vi "Teleop.vi"(10 "Match Info":T2={"Autonomous Elapsed Seconds"=0.0, "TeleOp Elapsed Seconds"=0.0, "Disabled Elapsed Seconds"=0.0, "Visited Autonomous"=FALSE, "Visited TeleOp"=FALSE, "Visited Disabled"=FALSE, "Autonomous Settings"={"Autonomous Style"=enum."Independent", "VI Refnum"=refnum}}, 11 "Call Context":T3) -> ()   [LabVIEW 2017]
doc: "This VI is called for each enabled TeleOp packet received from the DS. It is typically used to read from joysticks and other inputs and update I/O or setpoints for timed control loops. It should complete and return within 20 milliseconds or risk missing DS packets."
uses:
  <vilib>/Rock Robotics/WPI/DriverStation/WPI_DriverStationDerivedRobotMode.ctl
  <vilib>/Rock Robotics/WPI/DriverStation/WPI_DriverStationMatch Info.ctl
  Framework/Robot Global Data.vi
panel:
  in  "Tab Control":T1(tab)
  out "X_AxisCmd":dbl(graph)
  out "Y_AxisCmd":dbl(graph)
  out "RotationCmd":dbl(graph)
  out "DriveMotors":dbl[](graph)
  out "LiftMotorCmd":dbl(graph)
  out "ArmLiftMotorCmd":dbl(graph)
  out "Lift Max Limit":bool
  out "Lift Min Limit":bool
  out "Arm Lift Max Limit":bool
  out "Arm Lift Min Limit":bool
  out "RightArmMotorCmd":dbl(graph)
  out "LeftArmMotorCmd":dbl(graph)
  out "Right Arm Max Limit":bool
  out "Right Arm Min Limit":bool
  out "Left Arm Max Limit":bool
  out "Left Arm Min Limit":bool
  out "SqueezeMotorCmd":dbl(graph)
  out "HandMotorsCmd":dbl(graph)
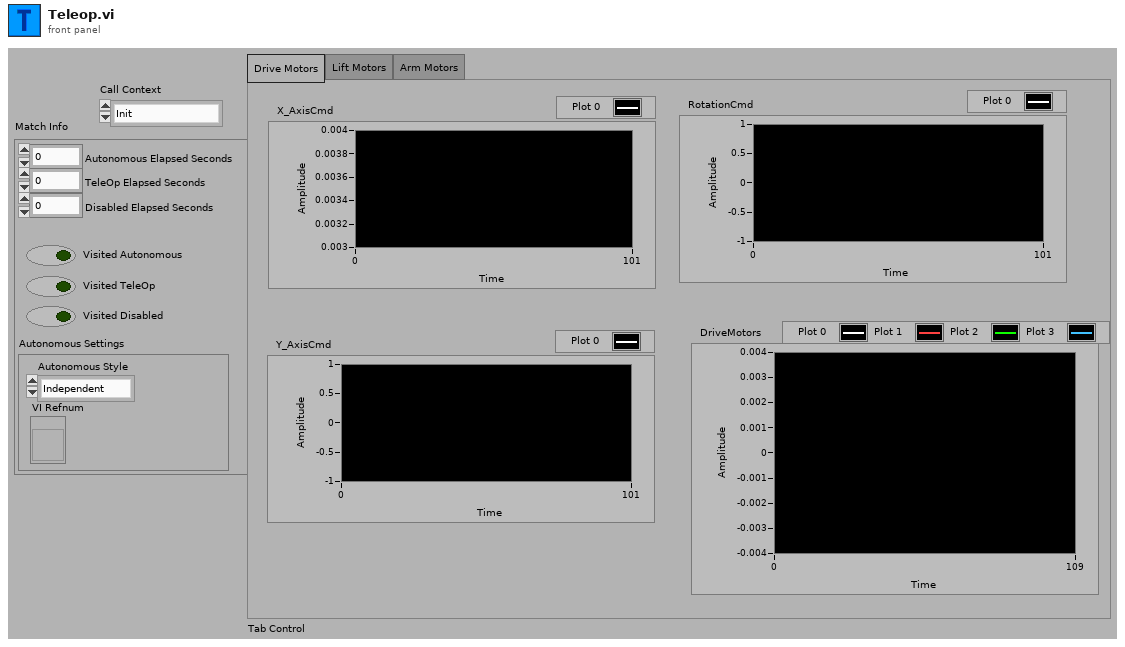
[diagram p1: front panel]
types:
  T1 = enum32{"Drive Motors", "Lift Motors", "Arm Motors"}
  T2 = typedef "WPI_DriverStationMatch Info.ctl" = cluster{"Autonomous Elapsed Seconds":dbl, "TeleOp Elapsed Seconds":dbl, "Disabled Elapsed Seconds":dbl, "Visited Autonomous":bool, "Visited TeleOp":bool, "Visited Disabled":bool, "Autonomous Settings":cluster{"Autonomous Style":enum16{"Iterative", "Independent"}, "VI Refnum":refnum<vi>}}
  T3 = typedef "WPI_DriverStationDerivedRobotMode.ctl" = enum16{"Init", "Execute", "Stop"}
  T4 = enum16{"initialize", "read", "write", "write all"}
  T5 = typedef "Joystick_XBox_0_Data.ctl" = cluster{"LX_Axis":dbl, "LY_Axis":dbl, "LTrigger_Axis":dbl, "RTrigger_Axis":dbl, "RX_Axis":dbl, "RY_Axis":dbl, "Button_0":bool, "Button_1":bool, "Button_2":bool, "Button_3":bool, "Button_4":bool, "Button_5":bool, "Button_6":bool, "Button_7":bool, "Button_8":bool, "Button_9":bool, "POV_0":i16, "POV_1":i16}
  T6 = typedef "Joystick_Generic_0_Data.ctl" = cluster{"X_Axis":dbl, "Y_axis":dbl, "Z_Axis":dbl, "Axis_3":dbl, "Axis_4":dbl, "Axis_5":dbl, "Button_0":bool, "Button_1":bool, "Button_2":bool, "Button_3":bool, "Button_4":bool, "Button_5":bool, "Button_6":bool, "Button_7":bool, "Button_8":bool, "Button_9":bool}
  T7 = typedef "WPI_SwitchDevRef.ctl" = cluster{"DevStatus":errorcluster, "DIO Channel":T8, "CntIndex":T9, "Normally Closed":bool}
  T8 = typedef "FPGA_DIOChannel.ctl" = enum8{"DIO 0", "DIO 1", "DIO 2", "DIO 3", "DIO 4", "DIO 5", "DIO 6", "DIO 7", "DIO 8", "DIO 9", "DIO MXP 0", "DIO MXP 1", "DIO MXP 2", "DIO MXP 3", "DIO MXP 4", "DIO MXP 5", "DIO MXP 6", "DIO MXP 7", "DIO MXP 8", "DIO MXP 9", "DIO MXP 10", "DIO MXP 11", "DIO MXP 12", "DIO MXP 13", "DIO MXP 14", "DIO MXP 15", "SPI Port CS1", "SPI Port CS2", "SPI Port CS3", "SPI Port MISO", "SPI Port MOSI", "Invalid"}
  T9 = typedef "FPGA_CounterCtrSystemIndex.ctl" = enum8{"Ctr 0", "Ctr 1", "Ctr 2", "Ctr 3", "Ctr 4", "Ctr 5", "Ctr 6", "Ctr 7", "Invalid"}
  T10 = typedef "DioDisplayALB.ctl" = cluster{"DIO 0-LiftMinLimitSwitch":bool, "DIO 1-LiftMaxLimitSwitch":bool, "DIO 2-LiftArmMinLimitSwitch":bool, "DIO 3-LiftArmMaxLimitSwitch":bool, "DIO 4-RightArmMaxLimitSwitch":bool, "DIO 5-RightArmMinLimitSwitch":bool, "DIO 6-LeftArmMaxLimitSwitch":bool, "DIO 7-LeftArmMinLimitSwitch":bool, "DIO 8":bool, "DIO 9":bool}
  T11 = typedef "Gyro_TypeDef.ctl" = cluster{"Angle":dbl, "AngularRate":dbl, "Calibrated":bool}
  T12 = typedef "WPI_MotorControlDeviceRef.ctl" = cluster{"DeviceStatus":errorcluster, "Type":T13, "PWM":cluster{"PWM Channel":T14, "DeadBand":T15}, "CAN":cluster{"Device Number":u8, "SetOutput VI Ref":variant, "GetOutput VI Ref":variant, "Enable VI Ref":variant, "Disable VI Ref":variant, "Data":variant}, "Invert":bool, "DIO PWM":cluster{"PWM \"Enable\" Channel":T14, "DIOChannel":T8, "PWM Rate":dbl}}
  T13 = typedef "WPI_MotorControlType.ctl" = enum16{"PWM", "CAN", "DIO PWM"}
  T14 = typedef "FPGA_DIOPWMChannel.ctl" = enum8{"PWM 0", "PWM 1", "PWM 2", "PWM 3", "PWM 4", "PWM 5", "PWM 6", "PWM 7", "PWM 8", "PWM 9", "PWM MXP 0", "PWM MXP 1", "PWM MXP 2", "PWM MXP 3", "PWM MXP 4", "PWM MXP 5", "PWM MXP 6", "PWM MXP 7", "PWM MXP 8", "PWM MXP 9", "Invalid"}
  T15 = typedef "WPI_PWMDeadband.ctl" = cluster{"Name":string, "maxPositivePwm":i32, "minPositivePwm":i32, "centerPwm":i32, "maxNegativePwm":i32, "minNegativePwm":i32, "angularRange":u16}
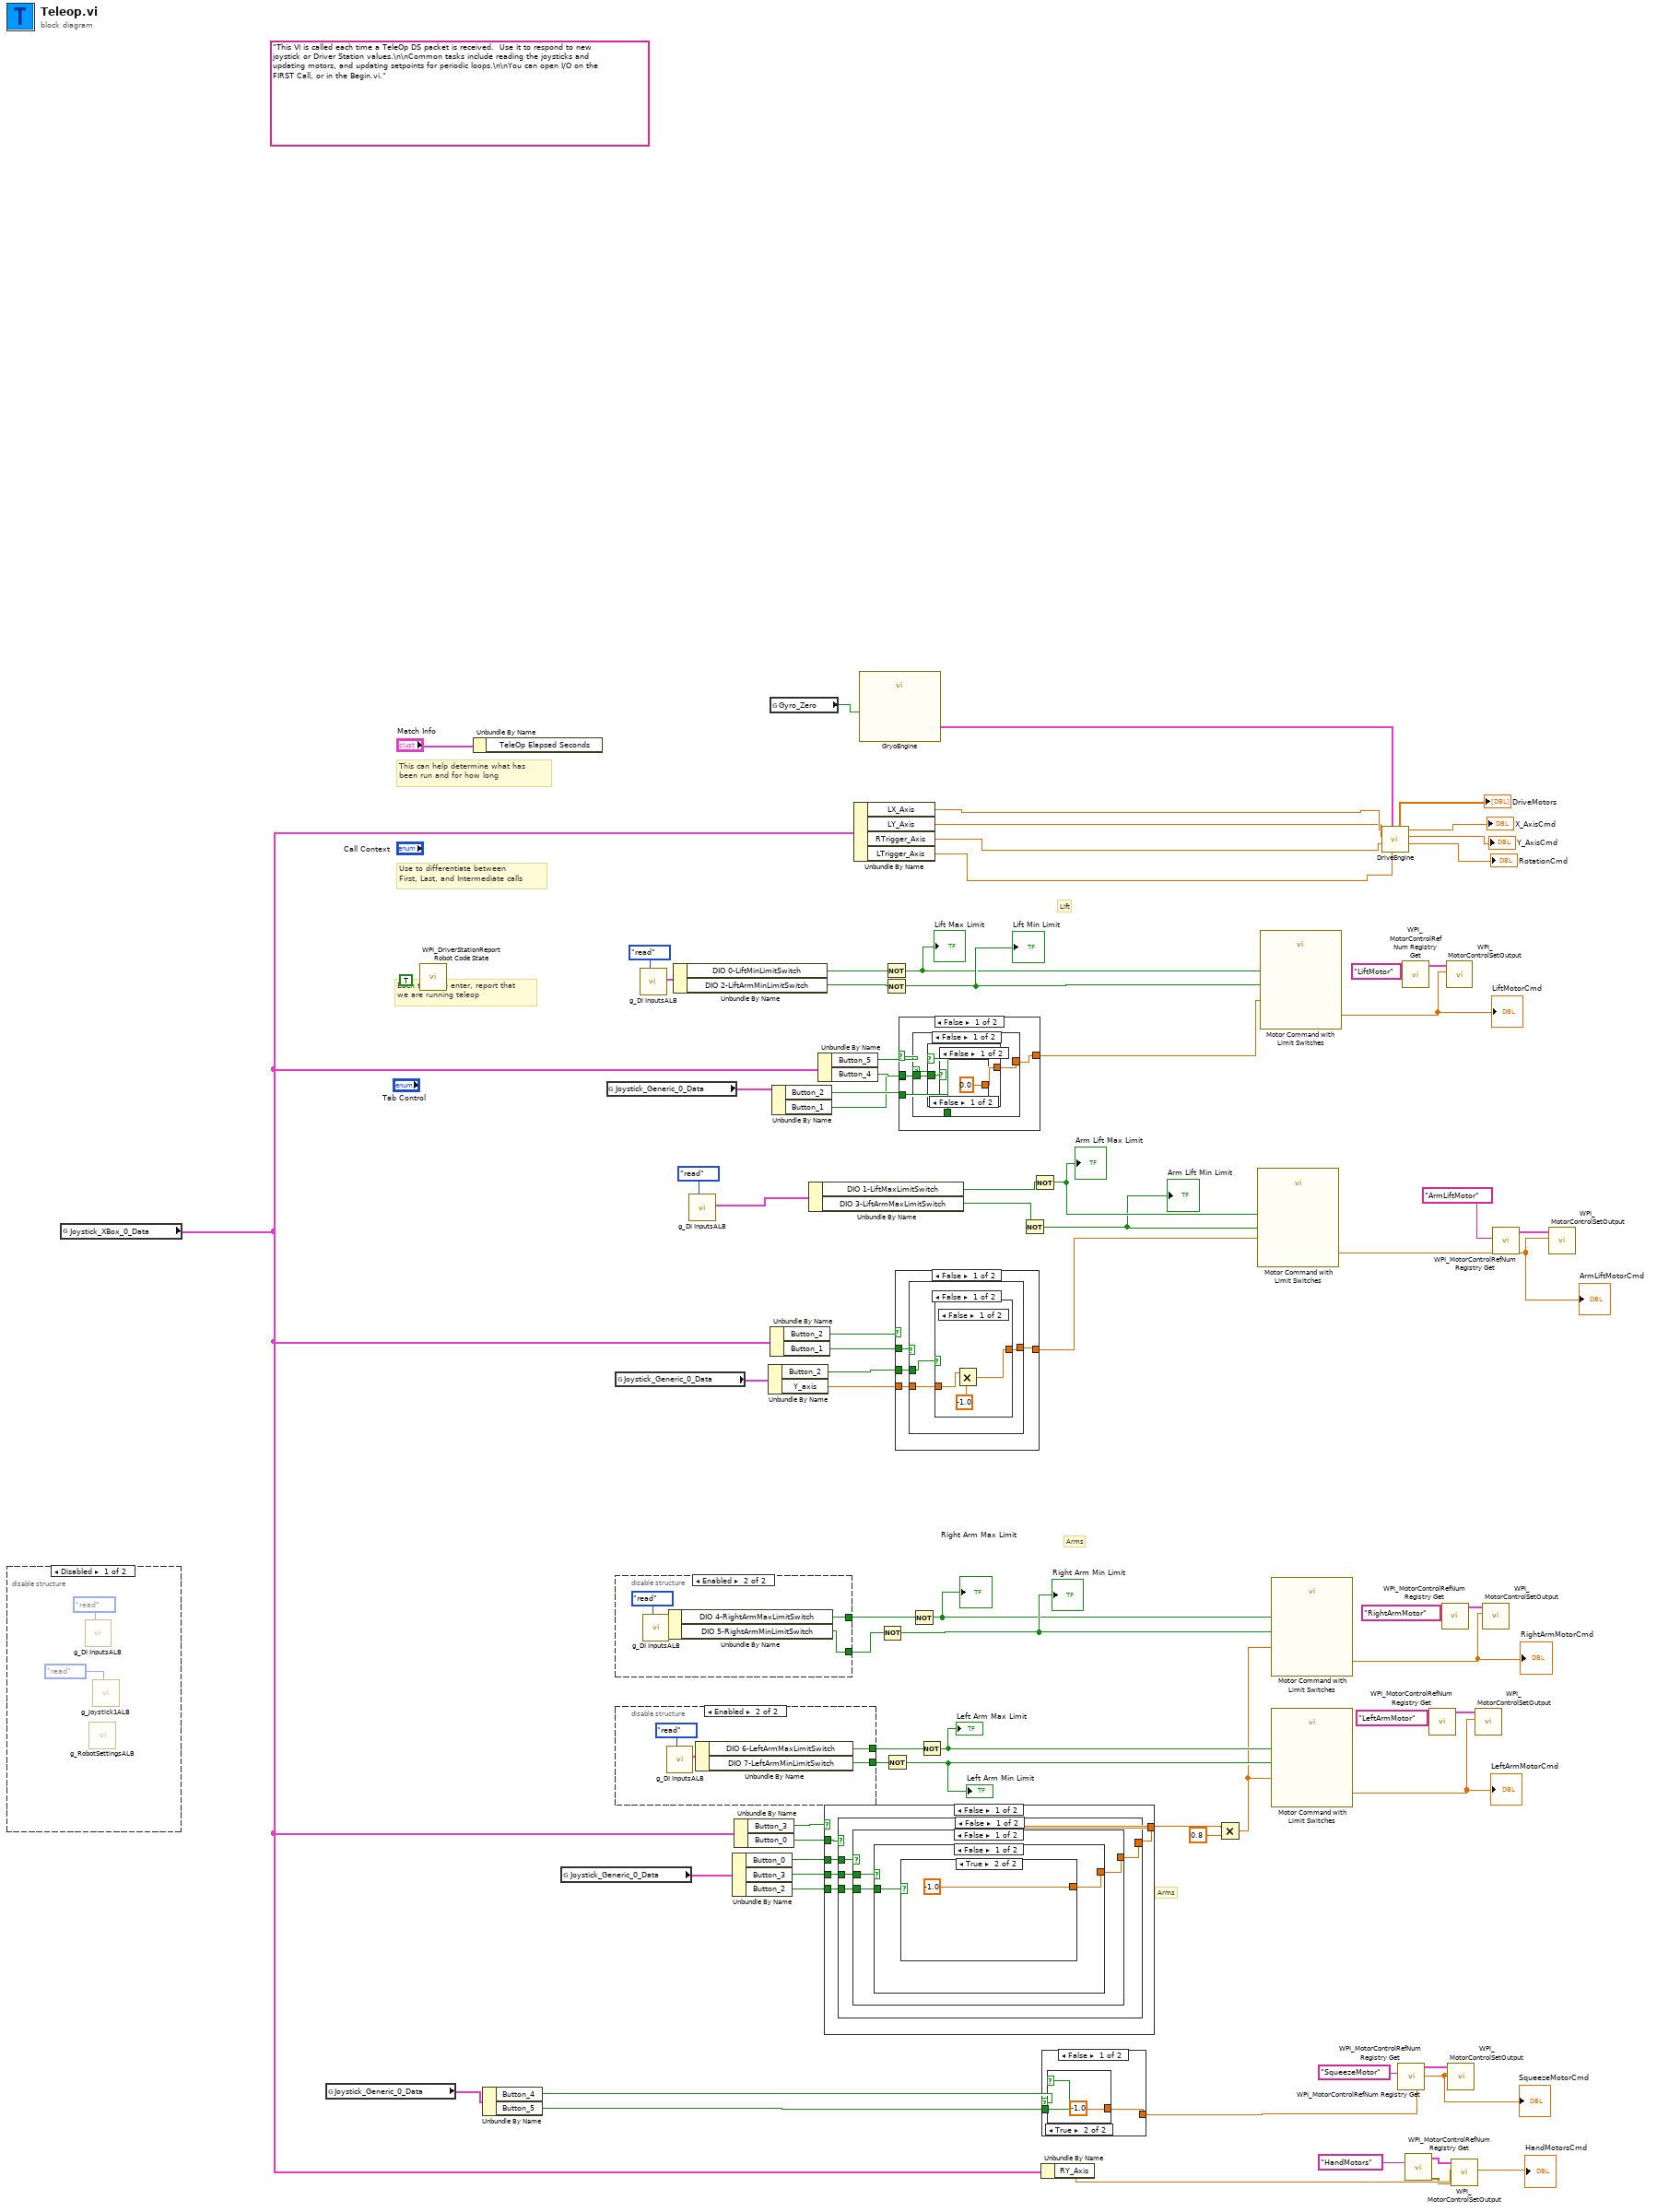
[diagram p0: block diagram]
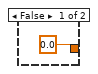
[diagram p2: hidden frame]
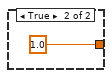
[diagram p3: hidden frame]
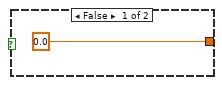
[diagram p4: hidden frame]
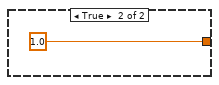
[diagram p5: hidden frame]
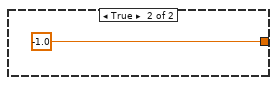
[diagram p6: hidden frame]
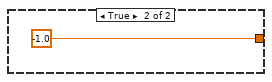
[diagram p7: hidden frame]
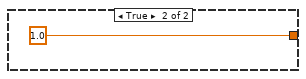
[diagram p8: hidden frame]
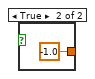
[diagram p9: hidden frame]
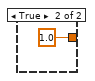
[diagram p10: hidden frame]
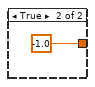
[diagram p11: hidden frame]
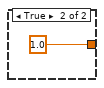
[diagram p12: hidden frame]
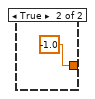
[diagram p13: hidden frame]
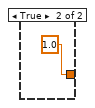
[diagram p14: hidden frame]
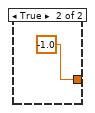
[diagram p15: hidden frame]
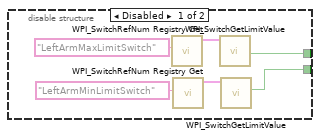
[diagram p17: hidden frame]
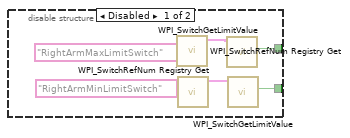
[diagram p18: hidden frame]
diagram:
  w66 = "SqueezeMotor"
  (unwired) "This VI is called each time a TeleOp DS packet is received.  Use it to respond to new joystick or Driver Station values.\n\nCommon tasks include reading the joysticks and updating motors, and updating setpoints for periodic loops.\n\nYou can open I/O on the FIRST Call, or in the Begin.vi."
  # "Arms"
  # "Arms"
  # "Lift"
  # "Each time we enter, report that\nwe are running teleop"
  # "Use to differentiate between\nFirst, Last, and Intermediate calls"
  # "This can help determine what has\nbeen run and for how long"
  n1 = disable-structure shown="Disabled" {
    frame Disabled {
      n2 = call "g_DI InputsALB.vi"("Action"=T4."read") -> ()  [unwired: 10 in, 1 out]
      n3 = call "g_RobotSettingsALB.vi"() -> ()  [unwired: 11 in, 1 out]
      n4 = call "g_Joystick1ALB.vi"("Action"=enum16{"initialize", "read", "write"}."read") -> ()  [unwired: 7 in, 4 out]
    }
    frame Enabled {
    }
  }
  n5 = global read "Robot Global Data.vi" "Joystick_XBox_0_Data"() -> (w29:T5)
  n6 = global read "Robot Global Data.vi" "Joystick_Generic_0_Data"() -> (w23:T6)
  n7 = call <vilib>:"WPI_DriverStationReport Robot Code State.vi"("TeleOp"=TRUE ("Autonomous")) -> ()  [unwired: 10 in, 1 out]
  n8 = Unbundle By Name("Match Info") -> ()  [unwired: 1 out]
  n9 = Unbundle By Name(w23) -> ("Button_4"=w2:bool, "Button_5"=w1:bool)
  n10 = global read "Robot Global Data.vi" "Joystick_Generic_0_Data"() -> (w22:T6)
  n11 = global read "Robot Global Data.vi" "Joystick_Generic_0_Data"() -> (w36:T6)
  n12 = global read "Robot Global Data.vi" "Joystick_Generic_0_Data"() -> (w43:T6)
  n13 = disable-structure shown="Enabled" {
    disable-tunnel: [w81 w86] -> w54
    disable-tunnel: [w80 w87] -> w53
    frame Disabled {
      n14 = call <vilib>:"WPI_SwitchRefNum Registry Get.vi"("refnum name"="RightArmMaxLimitSwitch") -> ("SwitchDevRef"=w84:T7)  [unwired: 9 in, 1 out]
      n15 = call <vilib>:"WPI_SwitchRefNum Registry Get.vi"("refnum name"="RightArmMinLimitSwitch") -> ("SwitchDevRef"=w83:T7)  [unwired: 9 in, 1 out]
      n16 = call <vilib>:"WPI_SwitchGetLimitValue.vi"("SwitchDevRef"=w84) -> ("Switch Pressed"=w80:bool)  [unwired: 8 in, 2 out]
      n17 = call <vilib>:"WPI_SwitchGetLimitValue.vi"("SwitchDevRef"=w83) -> ("Switch Pressed"=w81:bool)  [unwired: 8 in, 2 out]
    }
    frame Enabled {
      n18 = call "g_DI InputsALB.vi"("Action"=T4."read") -> ("DI out"=w88:T10)  [unwired: 10 in]
      n19 = Unbundle By Name(w88) -> ("DIO 4-RightArmMaxLimitSwitch"=w87:bool, "DIO 5-RightArmMinLimitSwitch"=w86:bool)
    }
  }
  n20 = disable-structure shown="Enabled" {
    disable-tunnel: [w91 w96] -> w56
    disable-tunnel: [w90 w97] -> w55
    frame Disabled {
      n21 = call <vilib>:"WPI_SwitchRefNum Registry Get.vi"("refnum name"="LeftArmMaxLimitSwitch") -> ("SwitchDevRef"=w95:T7)  [unwired: 9 in, 1 out]
      n22 = call <vilib>:"WPI_SwitchRefNum Registry Get.vi"("refnum name"="LeftArmMinLimitSwitch") -> ("SwitchDevRef"=w94:T7)  [unwired: 9 in, 1 out]
      n23 = call <vilib>:"WPI_SwitchGetLimitValue.vi"("SwitchDevRef"=w95) -> ("Switch Pressed"=w90:bool)  [unwired: 8 in, 2 out]
      n24 = call <vilib>:"WPI_SwitchGetLimitValue.vi"("SwitchDevRef"=w94) -> ("Switch Pressed"=w91:bool)  [unwired: 8 in, 2 out]
    }
    frame Enabled {
      n25 = call "g_DI InputsALB.vi"("Action"=T4."read") -> ("DI out"=w99:T10)  [unwired: 10 in]
      n26 = Unbundle By Name(w99) -> ("DIO 6-LeftArmMaxLimitSwitch"=w97:bool, "DIO 7-LeftArmMinLimitSwitch"=w96:bool)
    }
  }
  n27 = call "g_DI InputsALB.vi"("Action"=T4."read") -> ("DI out"=w19:T10)  [unwired: 10 in]
  n28 = Unbundle By Name(w19) -> ("DIO 0-LiftMinLimitSwitch"=w17:bool, "DIO 2-LiftArmMinLimitSwitch"=w16:bool)
  n29 = call "g_DI InputsALB.vi"("Action"=T4."read") -> ("DI out"=w20:T10)  [unwired: 10 in]
  n30 = Unbundle By Name(w22) -> ("Button_0"=w32:bool, "Button_3"=w12:bool, "Button_2"=w11:bool)
  n31 = Unbundle By Name(w29) -> ("Button_3"=w34:bool, "Button_0"=w33:bool)
  n32 = Unbundle By Name(w43) -> ("Button_2"=w40:bool, "Y_axis"=w13:dbl)
  n33 = global read "Robot Global Data.vi" "Gyro_Zero"() -> (w46:bool)
  n34 = Unbundle By Name(w29) -> ("Button_2"=w42:bool, "Button_1"=w31:bool)
  n35 = Unbundle By Name(w36) -> ("Button_2"=w35:bool, "Button_1"=w7:bool)
  n36 = Unbundle By Name(w20) -> ("DIO 1-LiftMaxLimitSwitch"=w15:bool, "DIO 3-LiftArmMaxLimitSwitch"=w14:bool)
  n37 = Unbundle By Name(w29) -> ("Button_5"=w39:bool, "Button_4"=w37:bool)
  n38 = case shown="False" w34 {
    tunnel: [w103 1.0] -> w10
    tunnel: w33 -> [w104 _]
    tunnel: w32 -> [w102 _]
    tunnel: w12 -> [w101 _]
    tunnel: w11 -> [w100 _]
    frame False {
      n39 = case shown="False" w104 {
        tunnel: [w108 -1.0] -> w103
        tunnel: w102 -> [w107 _]
        tunnel: w101 -> [w106 _]
        tunnel: w100 -> [w105 _]
        frame False {
          n40 = case shown="False" w107 {
            tunnel: [w110 -1.0] -> w108
            tunnel: w106 -> [w111 _]
            tunnel: w105 -> [w109 _]
            frame False {
              n41 = case shown="False" w111 {
                tunnel: [w112 1.0] -> w110
                tunnel: w109 -> [w113 _]
                frame False {
                  n42 = case shown="True" w113 {
                    tunnel: [0.0 -1.0] -> w112
                    frame False {
                    }
                    frame True {
                    }
                  }
                }
                frame True {
                }
              }
            }
            frame True {
            }
          }
        }
        frame True {
        }
      }
    }
    frame True {
    }
  }
  n43 = Unbundle By Name(w29) -> ("LX_Axis"=w6:dbl, "LY_Axis"=w5:dbl, "RTrigger_Axis"=w4:dbl, "LTrigger_Axis"=w3:dbl)
  n44 = call "GryoEngine.vi"("Gyro_Zero"=w46) -> ("GyroData"=w44:T11)  [unwired: 10 in]
  n45 = Not(x=w54) -> (.not. x?=w50:bool)
  "Right Arm Min Limit" <- w50
  n46 = Not(x=w17) -> (.not. x?=w59:bool)
  "Lift Max Limit" <- w59
  n47 = Not(x=w16) -> (.not. x?=w60:bool)
  "Lift Min Limit" <- w60
  n48 = Not(x=w56) -> (.not. x?=w48:bool)
  "Left Arm Min Limit" <- w48
  n49 = case shown="False" w42 {
    tunnel: [w121 -1.0] -> w41
    tunnel: w40 -> [w123 _]
    tunnel: w31 -> [w122 _]
    tunnel: w13 -> [w120 _]
    frame False {
      n50 = case shown="False" w122 {
        tunnel: [w126 1.0] -> w121
        tunnel: w123 -> [w125 _]
        tunnel: w120 -> [w124 _]
        frame False {
          n51 = case shown="False" w125 {
            tunnel: [w127 -1.0] -> w126
            tunnel: w124 -> [w129 _]
            frame False {
              n52 = Multiply(x=w129, y=-1.0) -> (x*y=w127:dbl)
            }
            frame True {
            }
          }
        }
        frame True {
        }
      }
    }
    frame True {
    }
  }
  n53 = case shown="False" w39 {
    tunnel: [w135 1.0] -> w38
    tunnel: w37 -> [w136 _]
    tunnel: w35 -> [w134 _]
    tunnel: w7 -> [w133 _]
    frame False {
      n54 = case shown="False" w136 {
        tunnel: [w139 -1.0] -> w135
        tunnel: w134 -> [w138 _]
        tunnel: w133 -> [w137 _]
        frame False {
          n55 = case shown="False" w138 {
            tunnel: [w140 1.0] -> w139
            tunnel: w137 -> [w141 _]
            frame False {
              n56 = case shown="False" w141 {
                tunnel: [0.0 -1.0] -> w140
                frame False {
                }
                frame True {
                }
              }
            }
            frame True {
            }
          }
        }
        frame True {
        }
      }
    }
    frame True {
    }
  }
  n57 = Not(x=w53) -> (.not. x?=w49:bool)
  "Right Arm Max Limit" <- w49
  n58 = Not(x=w55) -> (.not. x?=w47:bool)
  "Left Arm Max Limit" <- w47
  n59 = Not(x=w14) -> (.not. x?=w57:bool)
  "Arm Lift Min Limit" <- w57
  n60 = Not(x=w15) -> (.not. x?=w58:bool)
  "Arm Lift Max Limit" <- w58
  n61 = Unbundle By Name(w29) -> ("RY_Axis"=w27:dbl)
  n62 = case shown="False" w2 {
    tunnel: [w147 1.0] -> w30
    tunnel: w1 -> [w148 _]
    frame False {
      n63 = case shown="True" w148 {
        tunnel: [0.0 -1.0] -> w147
        frame False {
        }
        frame True {
        }
      }
    }
    frame True {
    }
  }
  "SqueezeMotorCmd" <- w30
  n64 = Multiply(x=w10, y=0.8) -> (x*y=w9:dbl)
  n65 = call "Motor Command with Limit Switches.vi"("LowLimitSwitch"=w57, "MotorCommandIn"=w41, "HighLimitSwitch"=w58) -> (0:w61:dbl)
  "ArmLiftMotorCmd" <- w61
  n66 = call "Motor Command with Limit Switches.vi"("LowLimitSwitch"=w60, "MotorCommandIn"=w38, "HighLimitSwitch"=w59) -> (0:w62:dbl)
  "LiftMotorCmd" <- w62
  n67 = call "Motor Command with Limit Switches.vi"("LowLimitSwitch"=w50, "MotorCommandIn"=w9, "HighLimitSwitch"=w49) -> (0:w52:dbl)
  "RightArmMotorCmd" <- w52
  n68 = call "Motor Command with Limit Switches.vi"("LowLimitSwitch"=w48, "MotorCommandIn"=w9, "HighLimitSwitch"=w47) -> (0:w51:dbl)
  "LeftArmMotorCmd" <- w51
  n69 = call "DriveEngine.vi"("RTrigger_Axis"=w3, "GyroData"=w44, "LTrigger_Axis"=w4, "LY_Axis"=w5, "LX_Axis"=w6) -> ("RotationCmd"=→"RotationCmd":dbl, "Y_AxisCmd"=→"Y_AxisCmd":dbl, "X_AxisCmd"=→"X_AxisCmd":dbl, "Motor Values"=→"DriveMotors":dbl[])  [unwired: 2 in, 1 out]
  n70 = call <vilib>:"WPI_MotorControlRefNum Registry Get.vi"("refnum name"=w66) -> ()  [unwired: 9 in, 2 out]
  n71 = call <vilib>:"WPI_MotorControlRefNum Registry Get.vi"("refnum name"=w66) -> ("MotorControlDevRef"=w67:T12)  [unwired: 9 in, 1 out]
  n72 = call <vilib>:"WPI_MotorControlRefNum Registry Get.vi"("refnum name"="LiftMotor") -> ("MotorControlDevRef"=w74:T12)  [unwired: 9 in, 1 out]
  n73 = call <vilib>:"WPI_MotorControlRefNum Registry Get.vi"("refnum name"="HandMotors") -> ("error out"=w26:errorcluster, "MotorControlDevRef"=w25:T12)  [unwired: 9 in]
  n74 = call <vilib>:"WPI_MotorControlRefNum Registry Get.vi"("refnum name"="LeftArmMotor") -> ("MotorControlDevRef"=w70:T12)  [unwired: 9 in, 1 out]
  n75 = call <vilib>:"WPI_MotorControlRefNum Registry Get.vi"("refnum name"="RightArmMotor") -> ("MotorControlDevRef"=w71:T12)  [unwired: 9 in, 1 out]
  n76 = call <vilib>:"WPI_MotorControlSetOutput.vi"("Output"=w62, "MotorControlDevRef"=w74) -> ()  [unwired: 7 in, 3 out]
  n77 = call <vilib>:"WPI_MotorControlSetOutput.vi"("Output"=w30, "MotorControlDevRef"=w67) -> ()  [unwired: 7 in, 3 out]
  n78 = call <vilib>:"WPI_MotorControlSetOutput.vi"("error in (no error)"=w26, "Output"=w27, "MotorControlDevRef"=w25) -> ("Motor Output"=→"HandMotorsCmd":dbl)  [unwired: 6 in, 2 out]
  n79 = call <vilib>:"WPI_MotorControlSetOutput.vi"("Output"=w51, "MotorControlDevRef"=w70) -> ()  [unwired: 7 in, 3 out]
  n80 = call <vilib>:"WPI_MotorControlSetOutput.vi"("Output"=w52, "MotorControlDevRef"=w71) -> ()  [unwired: 7 in, 3 out]
  n81 = call <vilib>:"WPI_MotorControlRefNum Registry Get.vi"("refnum name"="ArmLiftMotor") -> ("MotorControlDevRef"=w72:T12)  [unwired: 9 in, 1 out]
  n82 = call <vilib>:"WPI_MotorControlSetOutput.vi"("Output"=w61, "MotorControlDevRef"=w72) -> ()  [unwired: 7 in, 3 out]
